vi "WAV file reader.vi"() -> ()   [LabVIEW 2018]
uses:
  <vilib>/sound2/lvsound2.llb/Sound File Read Open.vi
  <vilib>/sound2/lvsound2.llb/Sound File Read (DBL).vi
panel:
  out "data":waveform(dbl)[](array[waveform])
  in  "path":path
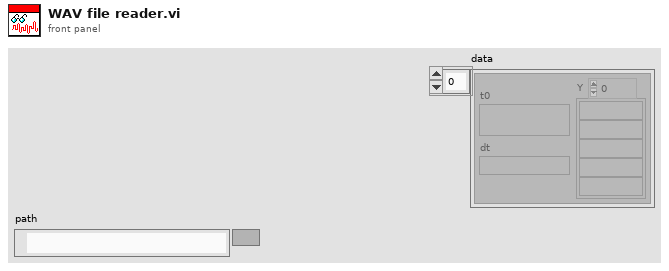
[diagram p1: front panel]
types:
  T1 = typedef "Sound File Refnum.ctl" = refnum<file>
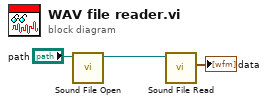
[diagram p0: block diagram]
diagram:
  n1 = call-poly <vilib>:"Sound File Open.vi"("path"="path") -> ("sound file refnum"=w2:T1)  [unwired: 9 in, 1 out]
  n2 = call-poly <vilib>:"Sound File Read.vi"("sound file refnum"=w2) -> ("data"=→"data":waveform(dbl)[])  [unwired: 6 in, 4 out]
